vi "Snap to bottom.vi"(8 "centered? (F)":bool, 9 "Fixed Rect":T1, 11 "Rect":T1) -> (1 "TopLeft point":cluster{"x":i32, "y":i32}, 3 "Snapped to bottom":T1)   [LabVIEW 2012]
doc: "This VI calculates the position of a snapped-to-bottom rectangle from the positions of a large rectangle and a smaller one that will be positioned inside."
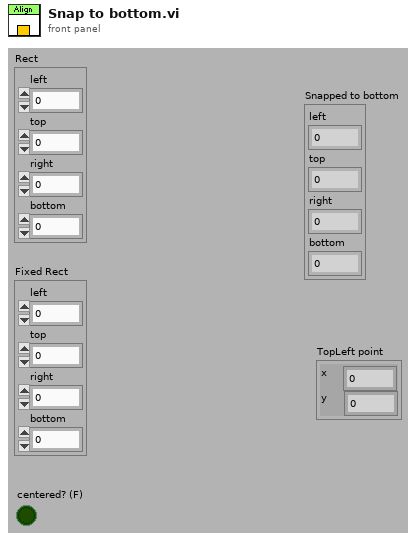
[diagram p1: front panel]
types:
  T1 = cluster{"left":i16, "top":i16, "right":i16, "bottom":i16}
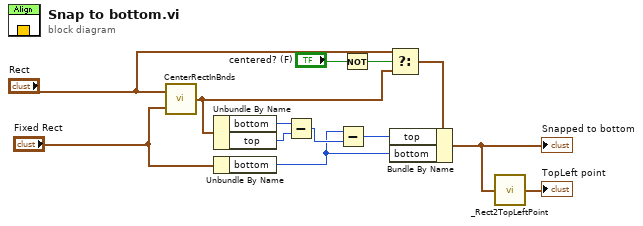
[diagram p0: block diagram]
diagram:
  n1 = call <vilib>:"CenterRectInBnds.vi"("bounds"="Fixed Rect", "rect"="Rect") -> ("centered rect"=w2:T1)
  n2 = Unbundle By Name(w2) -> ("bottom"=w8:i16, "top"=w9:i16)
  n3 = Unbundle By Name("Fixed Rect") -> ("bottom"=w7:i16)
  n4 = Subtract(x=w8, y=w9) -> (x-y=w10:i16)
  n5 = Subtract(x=w7, y=w10) -> (x-y=w6:i16)
  n6 = Not(x="centered? (F)") -> (.not. x?=w4:bool)
  n7 = Select(t="Rect", s=w4, f=w2) -> (s? t:f=w1:T1)
  n8 = Bundle By Name(cluster=w1, "top"=w6, "bottom"=w7) -> (w12:T1)
  "Snapped to bottom" <- w12
  n9 = call "_Rect2TopLeftPoint.vi"("bounds"=w12) -> ("TopLeft point"=→"TopLeft point":cluster{"x":i32, "y":i32})  [unwired: 4 out]
